vi "Live window-Ini.vi"(11 "Live img window ctrl refs":T1) -> (0 "error out":errorcluster, 2 "Queue timeout":i32=250, 3 "queue out":T3, 4 "Front Panel":refnum<vi>, 5 "Frame size":u16)   [LabVIEW 2017]
uses:
  Typedefs/Live graph data queue ref.ctl
  Queue/Live graphs queue/Typedefs/Live imaging queue element.ctl
  <vilib>/vision/Image Controls.llb/IMAQ Image.ctl
  Typedefs/Live window-ctrl refs.ctl
  Typedefs/Channel Selector.ctl
  Typedefs/Image display ref.ctl
  Typedefs/Save-Load enum.ctl
  Typedefs/Left-Right enum.ctl
  <vilib>/Utility/miscctls.llb/LVPointTypeDef.ctl
  Globals/gl_Windows Ctrl refs.vi
  Global Variables/General Globals.vi
  Global Variables/gl_UI Ctrl Refs.vi
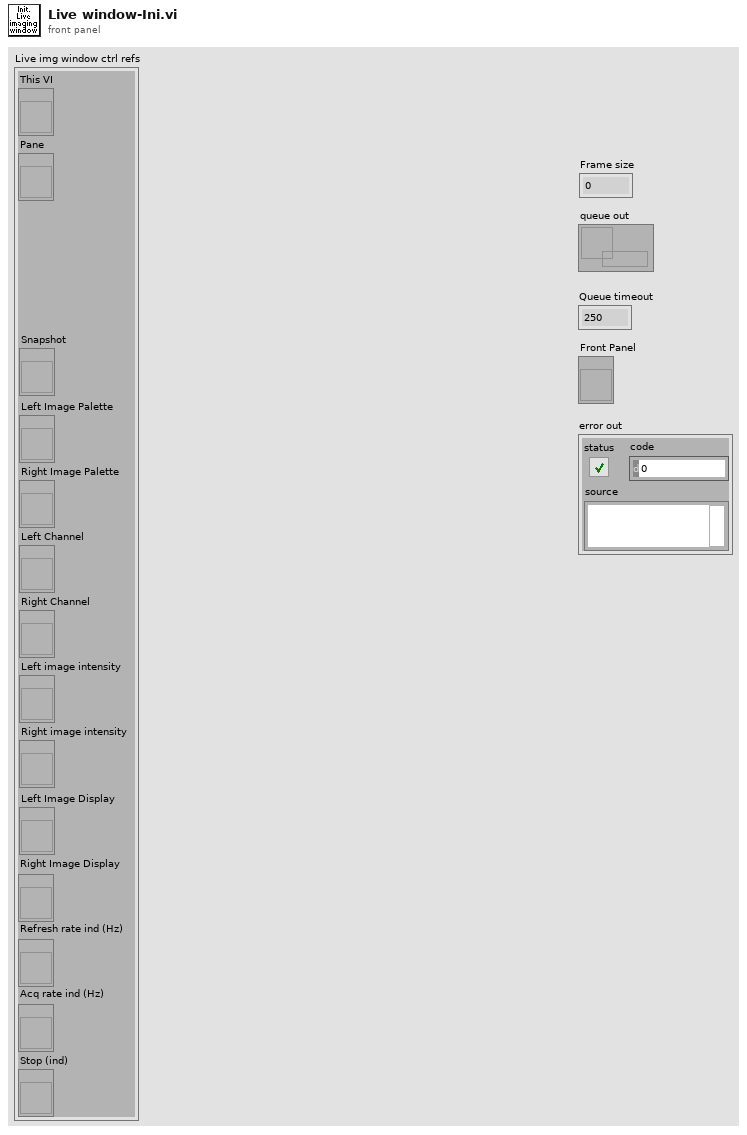
[diagram p1: front panel]
types:
  T1 = typedef "Live window-ctrl refs.ctl" = cluster{"This VI":refnum<vi>, "Pane":refnum<vi>, "Snapshot":refnum<vi>, "Left Image Palette":refnum<vi>, "Right Image Palette":refnum<vi>, "Left Channel":refnum<vi>, "Right Channel":refnum<vi>, "Left image intensity":refnum<vi>, "Right image intensity":refnum<vi>, "Left Image Display":T2, "Right Image Display":T2, "Refresh rate ind (Hz)":refnum<vi>, "Acq rate ind (Hz)":refnum<vi>, "Stop (ind)":refnum<vi>}
  T2 = typedef "Image display ref.ctl" = refnum<vi>
  T3 = typedef "Live graph data queue ref.ctl" = refnum<queue>
  T4 = typedef "Save-Load enum.ctl" = enum16{"Save to file", "Load from file", "Compare from file"}
  T5 = typedef "LVPointTypeDef.ctl" = cluster{"Horizontal":i16, "Vertical":i16}
  T6 = typedef "Left-Right enum.ctl" = enum16{"Right", "Left"}
  T7 = typedef "UI ctrl refs cluster.ctl" = cluster{"Top level VI path":path, "Top level VI ref":refnum<vi>, "User menu ref":refnum<k9>, "Sub Panel control":refnum<vi>, "Imaging Param Tab":refnum<vi>, "Occurrence-Start drivers":refnum<k4>, "Occurrence-Speed logging initialised":refnum<k4>, "Occurrence-XYZ stage initialised":refnum<k4>, "Exit button":refnum<vi>, "Status ind":refnum<vi>, "Set as origin":refnum<vi>, "Speed Logging":refnum<vi>, "Time Lapse":refnum<vi>, "Live Imaging":refnum<vi>, "AOL Z Stack":refnum<vi>, "Motor Z Stack":refnum<vi>, "Funct Acq button":refnum<vi>, "Hard Shutter":refnum<vi>, "Virtual Shutter":refnum<vi>, "Laser Power":refnum<vi>, "AOL Mode":refnum<vi>, "Frame Size":refnum<vi>, "Field of View":refnum<vi>, "Dwell Time":refnum<vi>, "Zoom":refnum<vi>, "AOL Z":refnum<vi>, "Objective":refnum<vi>, "Axis":refnum<vi>, "Paths & Names":refnum<vi>, "Experiment folder path (ind.)":refnum<vi>, "Last State (Ind.)":refnum<vi>, "Averages":refnum<vi>, "Angle (degrees)":refnum<vi>, "X centre":refnum<vi>, "Y centre":refnum<vi>, "Plane Mode":refnum<vi>, "# Planes":refnum<vi>, "Z Start":refnum<vi>, "Z Stop":refnum<vi>, "Z Step":refnum<vi>, "PMT 1":refnum<vi>, "PMT 2":refnum<vi>, "Stage XYZ Position":refnum<vi>, "Pockels@Z Start":refnum<vi>, "Pockels@Z Stop":refnum<vi>, "Obtain Z Start":refnum<vi>, "Obtain Z Stop":refnum<vi>, "Live stim.trig.period":refnum<vi>, "Live stim.trig.enable":refnum<vi>, "Funct. Acq. Pockels Modulation":refnum<vi>, "Enable Video Recording":refnum<vi>, "Video Record-Live Imaging":refnum<vi>, "Video Record-Funct acq":refnum<vi>, "AOL Z-stack Chirps Ready (ind)":refnum<vi>, "Center freq ind (nm)":refnum<vi>, "Logging queue (ind)":refnum<vi>, "Back aperture power (ind.)":refnum<vi>, "Power after objective (ind.)":refnum<vi>, "Switch user":refnum<vi>, "Ls1 Conn. Status":refnum<vi>, "Ls1Tuning Status":refnum<vi>, "Ls1 Faults":refnum<vi>, "Ls1 Connection":refnum<vi>, "Ls1 Mode":refnum<vi>, "Ls1 POWER [mW]":refnum<vi>, "Ls1Shutter":refnum<vi>, "Ls1 Wavelength":refnum<vi>, "Ls1 Note":refnum<vi>, "Ls1 Confirm Wav":refnum<vi>, "Ls1 PreChrp Prism1":refnum<vi>, "Ls1 PreChrp Prism2":refnum<vi>, "Ls1 wav top Ind":refnum<vi>, "Ls1 power top Ind":refnum<vi>, "Ls1 Pump peak Hold":refnum<vi>, "Ls1 Status Ind":refnum<vi>, "Ls1 wav cancel":refnum<vi>, "Experiment Type":refnum<vi>, "Biology Information":refnum<vi>}
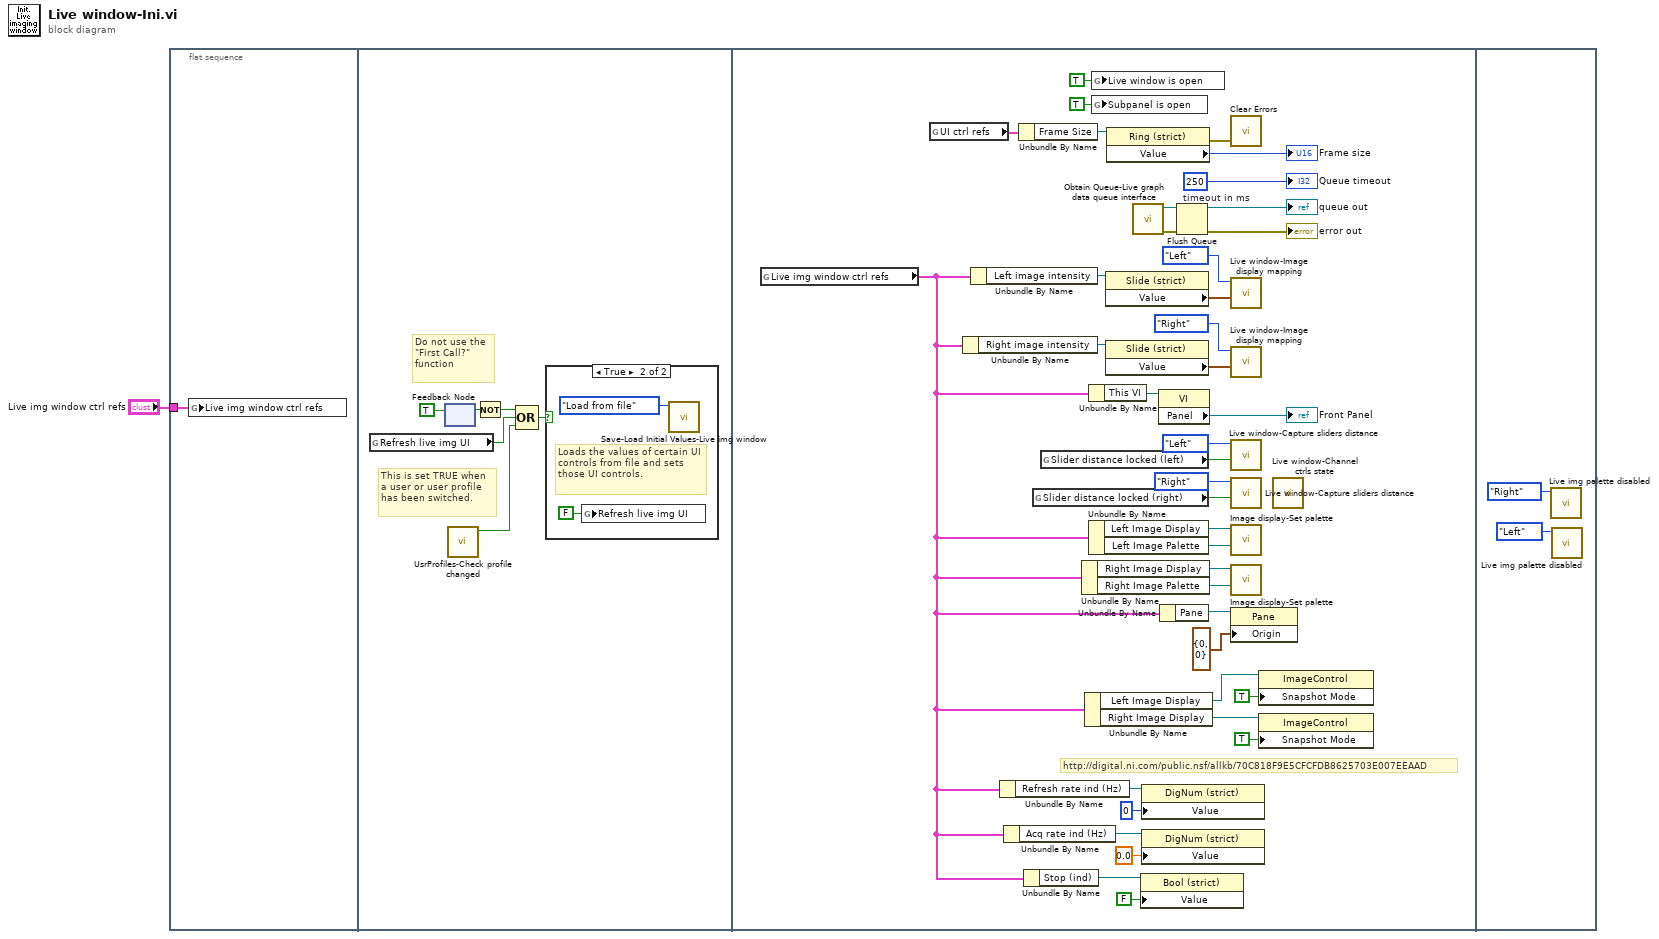
[diagram p0: block diagram]
diagram:
  n1 = flat-sequence {
    tunnel: "Live img window ctrl refs" -> [w2]
    frame #0 {
      n2 = global write "gl_Windows Ctrl refs.vi" "Live img window ctrl refs"(w2) -> ()
    }
    frame #1 {
      # "This is set TRUE when a user or user profile has been switched."
      # "Do not use the \"First Call?\" function"
      n3 = global read "gl_Windows Ctrl refs.vi" "Refresh live img UI"() -> (w4:bool)
      n4 = feedback #1() -> (w7:bool)  [unwired: 1 in]
      n5 = feedback-in #1(TRUE) -> ()
      n6 = call "UsrProfiles-Check profile changed.vi"() -> ("Profile changed"=w3:bool)  [unwired: 10 in, 1 out]
      n7 = Not(x=w7) -> (.not. x?=w6:bool)
      n8 = Compound Arithmetic op=OR(w6, w4, w3) -> (w5:bool)
      n9 = case shown="True" w5 {
        frame False {
        }
        frame True {
          # "Loads the values of certain UI controls from file and sets those UI controls."
          n10 = global write "gl_Windows Ctrl refs.vi" "Refresh live img UI"(FALSE ("Refresh live img UI")) -> ()
          n11 = call "Save-Load Initial Values-Live img window.vi"("Function"=Save-Load_enum."Load from file") -> ()  [unwired: 10 in, 1 out]
        }
      }
    }
    frame #2 {
      w33 = 250  # timeout in ms
      # "http://digital.ni.com/public.nsf/allkb/70C818F9E5CFCFDB8625703E007EEAAD"
      n12 = global read "gl_Windows Ctrl refs.vi" "Live img window ctrl refs"() -> (w12:T1)
      n13 = global read "gl_UI Ctrl Refs.vi" "UI ctrl refs"() -> (w40:T7)
      n14 = Unbundle By Name(w12) -> ("Right image intensity"=w24:refnum<vi>)
      n15 = Unbundle By Name(w12) -> ("Left image intensity"=w48:refnum<vi>)
      n16 = Unbundle By Name(w12) -> ("Refresh rate ind (Hz)"=w16:refnum<vi>)
      n17 = Unbundle By Name(w12) -> ("Acq rate ind (Hz)"=w17:refnum<vi>)
      n18 = Unbundle By Name(w40) -> ("Frame Size"=w41:refnum<vi>)
      n19 = Unbundle By Name(w12) -> ("Stop (ind)"=w13:refnum<vi>)
      n20 = global read "gl_Windows Ctrl refs.vi" "Slider distance locked (right)"() -> (w45:bool)
      n21 = global read "gl_Windows Ctrl refs.vi" "Slider distance locked (left)"() -> (w42:bool)
      n22 = Unbundle By Name(w12) -> ("Right Image Display"=w25:T2, "Right Image Palette"=w26:refnum<vi>)
      n23 = Unbundle By Name(w12) -> ("Left Image Display"=w21:T2, "Right Image Display"=w18:T2)
      n24 = Unbundle By Name(w12) -> ("This VI"=w32:refnum<vi>)
      n25 = Unbundle By Name(w12) -> ("Left Image Display"=w28:T2, "Left Image Palette"=w27:refnum<vi>)
      n26 = global write "General Globals.vi" "Live window is open"(TRUE ("Live window running")) -> ()
      n27 = global write "General Globals.vi" "Subpanel is open"(TRUE ("Subpanel is open")) -> ()
      n28 = property class="Slide (strict)"(reference=w48) -> ("Value"=w49:cluster{i16, i16})  [unwired: 1 in, 2 out]
      n29 = property class="Slide (strict)"(reference=w24) -> ("Value"=w50:cluster{i16, i16})  [unwired: 1 in, 2 out]
      n30 = property class="Ring (strict)"(reference=w41) -> (error out=w38:errorcluster, "Value"=→"Frame size":u16)  [unwired: 1 in, 1 out]
      n31 = call "Obtain Queue-Live graph data queue interface.vi"() -> ("error out"=w36:errorcluster, "Live graphs queue"=w37:T3)  [unwired: 10 in]
      n32 = property class="Bool (strict)"(reference=w13, "Value"=FALSE) -> ()  [unwired: 1 in, 2 out]
      n33 = property class="DigNum (strict)"(reference=w16, "Value"=0) -> ()  [unwired: 1 in, 2 out]
      n34 = property class="DigNum (strict)"(reference=w17, "Value"=0.0) -> ()  [unwired: 1 in, 2 out]
      n35 = property class="VI"(reference=w32) -> ("Panel"=→"Front Panel":refnum<vi>)  [unwired: 1 in, 2 out]
      n36 = Unbundle By Name(w12) -> ("Pane"=w22:refnum<vi>)
      n37 = Flush Queue(queue=w37, error in (no error)=w36) -> (queue out=→"queue out":T3, error out=→"error out":errorcluster)  [unwired: 1 out]
      n38 = call <vilib>:"Clear Errors.vi"("error in (no error)"=w38) -> ()  [unwired: 5 in, 2 out]
      n39 = call "Live window-Image display mapping.vi"("Intensity sliders"=w49, "Which image display?"=Left-Right_enum."Left") -> ()  [unwired: 9 in, 1 out]
      n40 = call "Live window-Image display mapping.vi"("Intensity sliders"=w50, "Which image display?"=Left-Right_enum."Right") -> ()  [unwired: 9 in, 1 out]
      n41 = call "Live window-Capture sliders distance.vi"("Locked?"=w42, "Function"=Left-Right_enum."Left") -> ()  [unwired: 10 in]
      n42 = call "Live window-Capture sliders distance.vi"("Locked?"=w45, "Function"=Left-Right_enum."Right") -> ()  [unwired: 10 in]
      n43 = call "Image display-Set palette.vi"("Image Palette"=w27, "Image Display"=w28) -> ()  [unwired: 8 in, 2 out]
      n44 = call "Image display-Set palette.vi"("Image Palette"=w26, "Image Display"=w25) -> ()  [unwired: 8 in, 2 out]
      n45 = property class="Pane"(reference=w22, "Origin"=T5 {"Horizontal"=0, "Vertical"=0}) -> ()  [unwired: 1 in, 2 out]
      n46 = property on="Property Node" class="ImageControl"(reference=w21, "Snapshot Mode"=TRUE) -> ()  [unwired: 1 in, 2 out]
      n47 = property on="Property Node" class="ImageControl"(reference=w18, "Snapshot Mode"=TRUE) -> ()  [unwired: 1 in, 2 out]
      n48 = call "Live window-Channel ctrls state.vi"() -> ()  [unwired: 12 in]
      "Queue timeout" <- w33
    }
    frame #3 {
      n49 = call "Live img palette disabled.vi"("Left/Right"=Left-Right_enum."Right") -> ()  [unwired: 10 in, 1 out]
      n50 = call "Live img palette disabled.vi"("Left/Right"=Left-Right_enum."Left") -> ()  [unwired: 10 in, 1 out]
    }
  }
